vi "Write Attributes.vi"(4 "Private":bool[](array[boolean]), 6 "Pointer":bool[](array[boolean]), 7 "Linked List ID":string, 8 "error in (no error)":errorcluster, 9 "Attributes":variant[](array[variant]), 10 "Attribute Names":string[](array[string]), 11 "Linked List in":refnum<class "Linked List.lvclass">) -> (0 "error out":errorcluster, 1 "Replaced?":bool[](array[boolean]), 2 "Unique IDs":string[](array[string]), 3 "Linked List out":refnum<class "Linked List.lvclass">)   [LabVIEW 2017, in "Linked Lists.lvlib" / "Linked List.lvclass"]
uses:
  <vilib>/gpm_packages/@cs/linked-list/Source/Linked List/Linked List/Linked List.lvclass
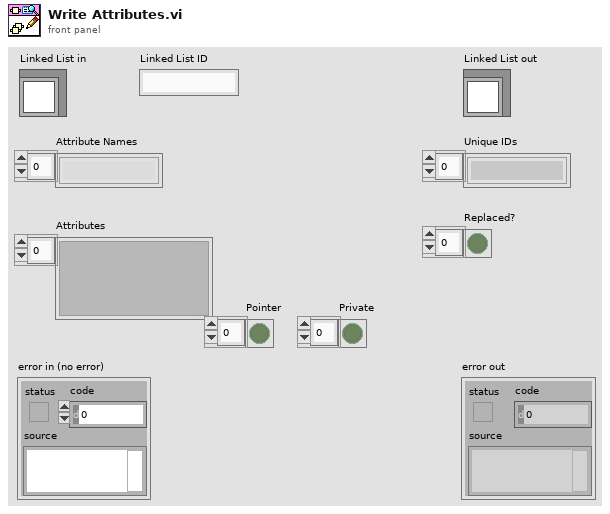
[diagram p1: front panel]
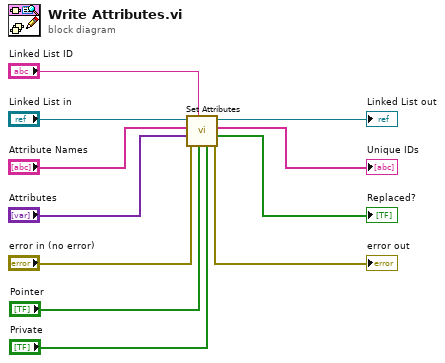
[diagram p0: block diagram]
diagram:
  n1 = call <vilib>:"Set Attributes.vi"("Private"="Private", "Pointer"="Pointer", "Unique ID"="Linked List ID", "error in (no error)"="error in (no error)", "Data"="Attributes", "Name"="Attribute Names", "Linked List in"="Linked List in") -> ("error out"=→"error out":errorcluster, "Replaced?"=→"Replaced?":bool[], "Unique IDs"=→"Unique IDs":string[], "Linked List out"=→"Linked List out":refnum<class "Linked List.lvclass">)  [unwired: 1 in]
